vi "CRYCheck Cal Curves for Load or Revert.vi"(8 "In_Out":bool, 9 "Calibration In":T1[](array[typedef]) {"Sens Curve"."Z data" items=["dB", "Lin"]; "Sens Curve"."X data" items=["dB", "Lin"]; "Sens Curve"."Y data" items=["dB", "Lin"]; "Sens Curve"."Z dB ref" format="%.1f"; "Sens Curve"."Z axis" items=["Log", "Lin"]; "Sens Curve"."X dB ref" format="%.1f"; "Sens Curve"."X axis" items=["Log", "Lin"]; "Sens Curve"."Y axis" items=["Log", "Lin"]; "Sens Curve"."Y dB ref" format="%.1f"; "Sens Curve"."Curve"."z" format="%.2f"; "Sens Curve"."Curve"."y" format="%.2f"; "Sens Curve"."Curve"."x" format="%.2f"; "EQ Curve"."Z data" items=["dB", "Lin"]; "EQ Curve"."X data" items=["dB", "Lin"]; "EQ Curve"."Y data" items=["dB", "Lin"]; "EQ Curve"."Z dB ref" format="%.1f"; "EQ Curve"."Z axis" items=["Log", "Lin"]; "EQ Curve"."X dB ref" format="%.1f"; "EQ Curve"."X axis" items=["Log", "Lin"]; "EQ Curve"."Y axis" items=["Log", "Lin"]; "EQ Curve"."Y dB ref" format="%.1f"; "EQ Curve"."Curve"."z" format="%.2f"; "EQ Curve"."Curve"."y" format="%.2f"; "EQ Curve"."Curve"."x" format="%.2f"; "Corr Curve"."Z data" items=["dB", "Lin"]; "Corr Curve"."X data" items=["dB", "Lin"]; "Corr Curve"."Y data" items=["dB", "Lin"]; "Corr Curve"."Z dB ref" format="%.1f"; "Corr Curve"."Z axis" items=["Log", "Lin"]; "Corr Curve"."X dB ref" format="%.1f"; "Corr Curve"."X axis" items=["Log", "Lin"]; "Corr Curve"."Y axis" items=["Log", "Lin"]; "Corr Curve"."Y dB ref" format="%.1f"; "Corr Curve"."Curve"."z" format="%.2f"; "Corr Curve"."Curve"."y" format="%.2f"; "Corr Curve"."Curve"."x" format="%.2f"; "Calibration"."EQ Step size" items=["R10", "R20", "R40", "R80", "User"]; "Calibration"."Corr Step size" items=["R10", "R20", "R40", "R80", "User"]}, 11 "Channel Info_New":T4[](array[typedef]) {"Coupling" items=["Default"=-1, "RSE"=10083, "NRSE"=10078, "Differential"=10106, "Pseudodifferential"=12529]; "term config" items=["Default"=-1, "RSE"=10083, "NRSE"=10078, "Differential"=10106, "Pseudodifferential"=12529]; "Anti-aliasing Factor (%fs)" format="%.2f"}) -> (3 "Calibration Out":T1[](array[typedef]) {"Sens Curve"."Z data" items=["dB", "Lin"]; "Sens Curve"."X data" items=["dB", "Lin"]; "Sens Curve"."Y data" items=["dB", "Lin"]; "Sens Curve"."Z dB ref" format="%.1f"; "Sens Curve"."Z axis" items=["Log", "Lin"]; "Sens Curve"."X dB ref" format="%.1f"; "Sens Curve"."X axis" items=["Log", "Lin"]; "Sens Curve"."Y axis" items=["Log", "Lin"]; "Sens Curve"."Y dB ref" format="%.1f"; "Sens Curve"."Curve"."z" format="%.2f"; "Sens Curve"."Curve"."y" format="%.2f"; "Sens Curve"."Curve"."x" format="%.2f"; "EQ Curve"."Z data" items=["dB", "Lin"]; "EQ Curve"."X data" items=["dB", "Lin"]; "EQ Curve"."Y data" items=["dB", "Lin"]; "EQ Curve"."Z dB ref" format="%.1f"; "EQ Curve"."Z axis" items=["Log", "Lin"]; "EQ Curve"."X dB ref" format="%.1f"; "EQ Curve"."X axis" items=["Log", "Lin"]; "EQ Curve"."Y axis" items=["Log", "Lin"]; "EQ Curve"."Y dB ref" format="%.1f"; "EQ Curve"."Curve"."z" format="%.2f"; "EQ Curve"."Curve"."y" format="%.2f"; "EQ Curve"."Curve"."x" format="%.2f"; "Corr Curve"."Z data" items=["dB", "Lin"]; "Corr Curve"."X data" items=["dB", "Lin"]; "Corr Curve"."Y data" items=["dB", "Lin"]; "Corr Curve"."Z dB ref" format="%.1f"; "Corr Curve"."Z axis" items=["Log", "Lin"]; "Corr Curve"."X dB ref" format="%.1f"; "Corr Curve"."X axis" items=["Log", "Lin"]; "Corr Curve"."Y axis" items=["Log", "Lin"]; "Corr Curve"."Y dB ref" format="%.1f"; "Corr Curve"."Curve"."z" format="%.2f"; "Corr Curve"."Curve"."y" format="%.2f"; "Corr Curve"."Curve"."x" format="%.2f"; "Calibration"."EQ Step size" items=["R10", "R20", "R40", "R80", "User"]; "Calibration"."Corr Step size" items=["R10", "R20", "R40", "R80", "User"]})   [LabVIEW 2013]
uses:
  Typedef Control/CRYCalibration 2DCluster.ctl
  Typedef Control/CRYCalibration Cluster.ctl
  Typedef Control/CRYData Cluster.ctl
  Typedef Control/CRYHardware Channel Info.ctl
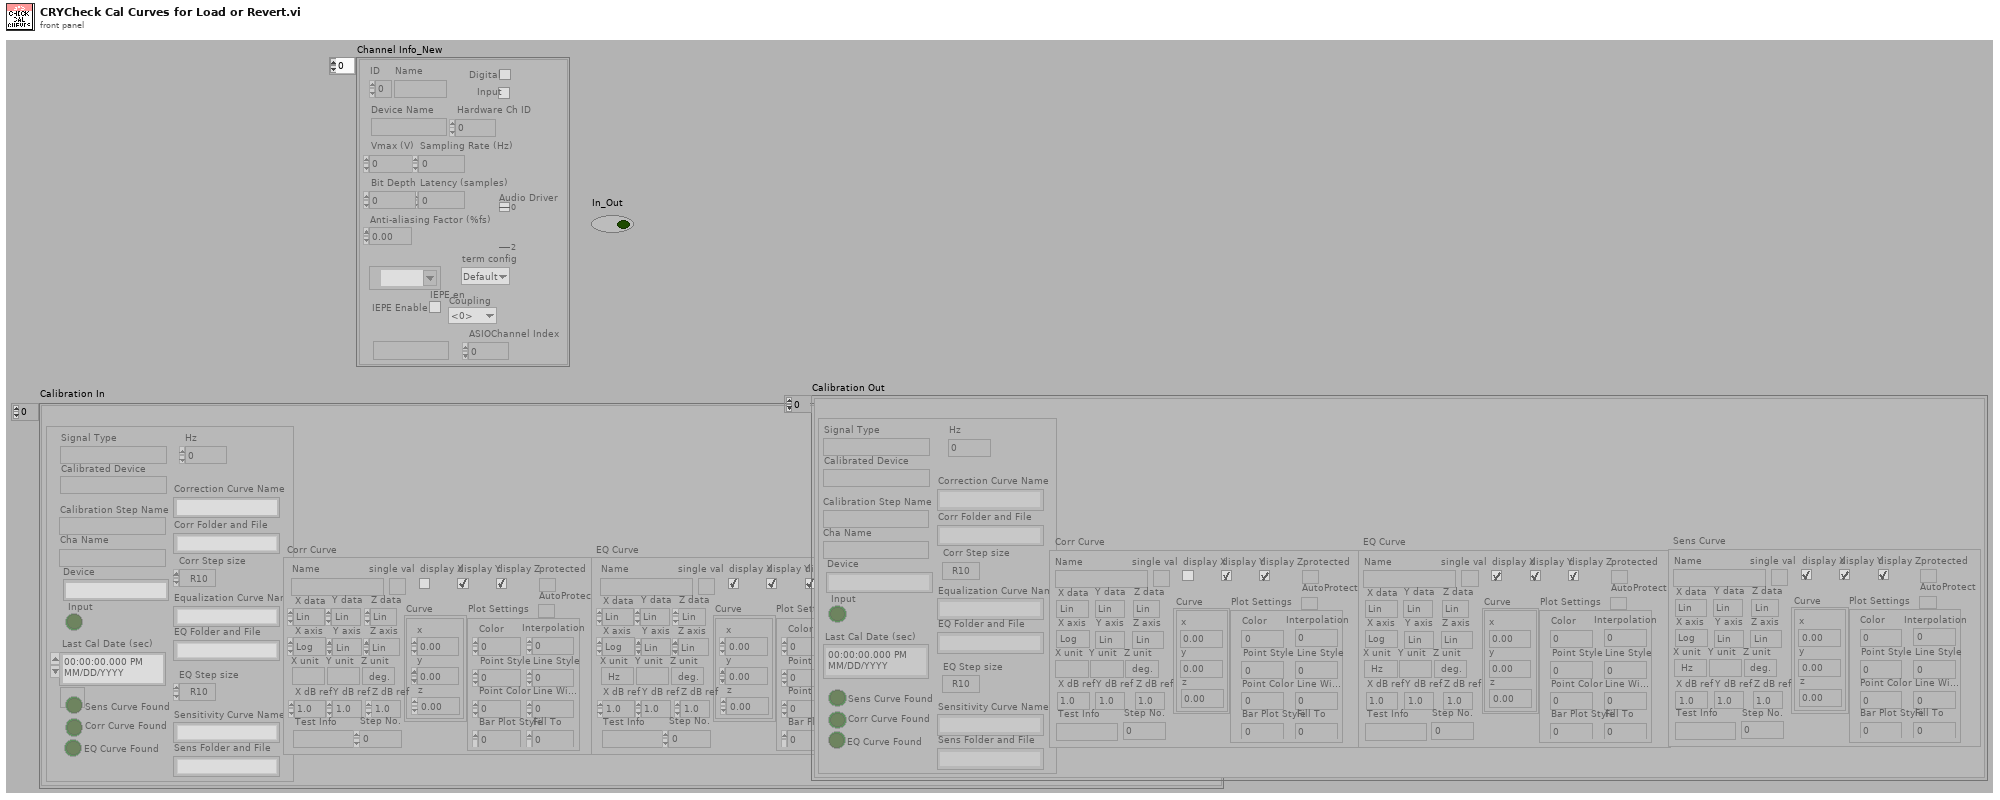
[diagram p1: front panel]
types:
  T1 = typedef "CRYCalibration 2DCluster.ctl" = cluster{"Calibration":T2, "Corr Curve":T3, "EQ Curve":T3, "Sens Curve":T3}
  T2 = typedef "CRYCalibration Cluster.ctl" = cluster{"Calibration Step Name":string, "Device":string, "Correction Curve Name":string, "Equalization Curve Name":string, "Sensitivity Curve Name":string, "Corr Folder and File":string, "EQ Folder and File":string, "Sens Folder and File":string, "Corr Step size":u16, "EQ Step size":u16, "Input":bool, "Last Cal Date (sec)":timestamp, "Cha Name":string, "Corr Curve Found":bool, "EQ Curve Found":bool, "Sens Curve Found":bool, "Signal Type":string, "Calibrated Device":string, "Hz":u32}
  T3 = typedef "CRYData Cluster.ctl" = cluster{"Name":string, "Curve":cluster{"x":dbl, "y":dbl, "z":dbl}[], "X data":u16, "Y data":u16, "Z data":u16, "X axis":u16, "Y axis":u16, "Z axis":u16, "X unit":string, "Y unit":string, "Z unit":string, "X dB ref":dbl, "Y dB ref":dbl, "Z dB ref":dbl, "single val":bool, "protected":bool, "display X":bool, "display Y":bool, "display Z":bool, "Test Info":string, "Step No.":i32, "Plot Settings":cluster{"Color":u32, "Interpolation":u8, "Point Style":u8, "Line Style":u8, "Point Color":u32, "Line Width":u8, "Bar Plot Style":u8, "Fill To":i16}, "AutoProtect":bool}
  T4 = typedef "CRYHardware Channel Info.ctl" = cluster{"ID":i32, "Name":string, "Digital":bool, "Input":bool, "Device Name":string, "Hardware Ch ID":u8, "Vmax (V)":dbl, "Latency (samples)":dbl, "Sampling Rate (Hz)":u32, "Bit Depth":u32, "Anti-aliasing Factor (%fs)":sgl, "DAQmx Channel":tag, "term config":i32, "Coupling":i32, "IEPE en":bool, "ASIOChannel Name":string, "Audio Driver":u16, "ASIOChannel Index":u8}
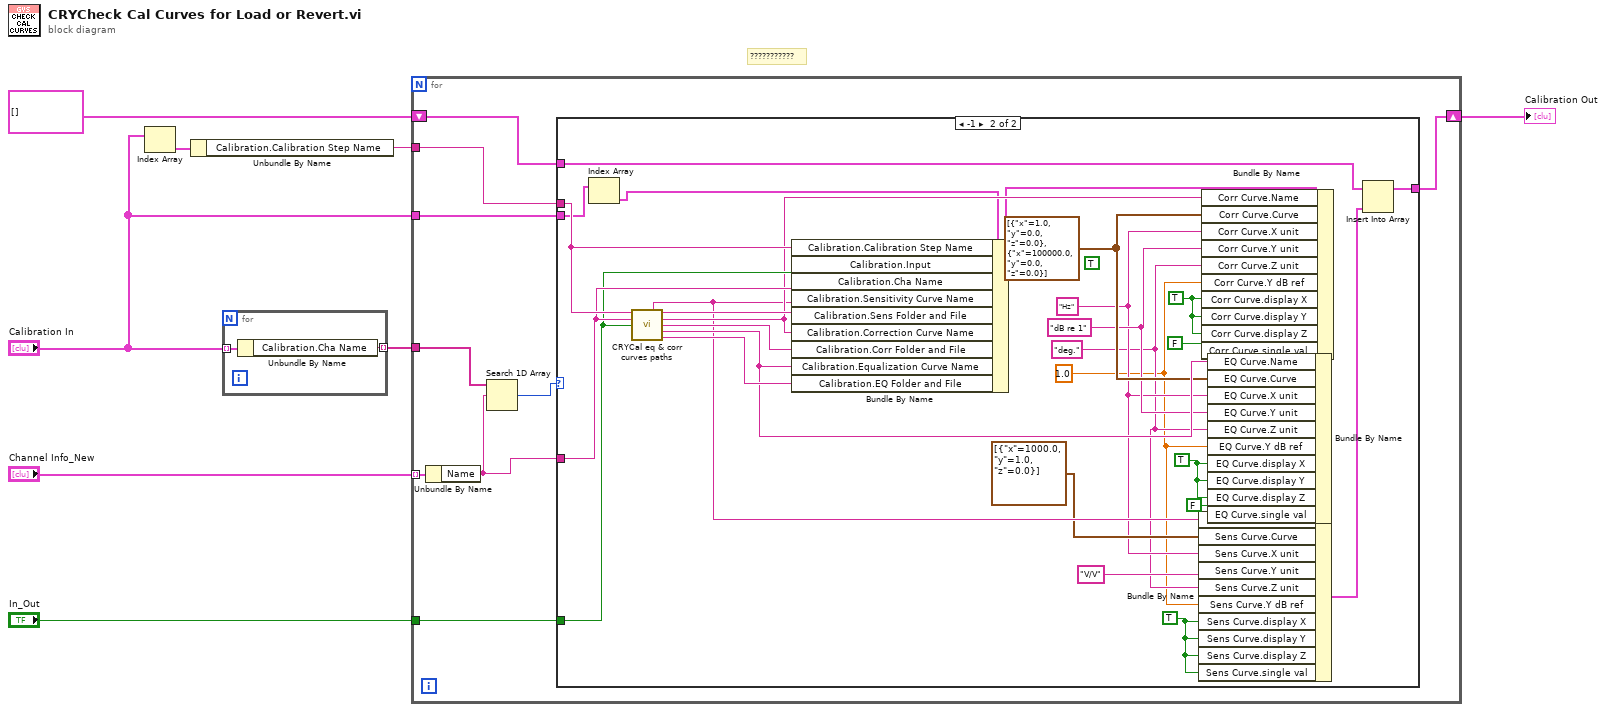
[diagram p0: block diagram]
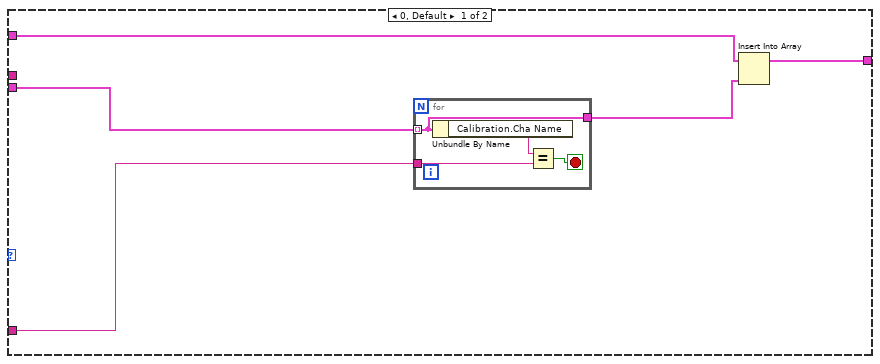
[diagram p2: hidden frame]
diagram:
  # "???????????"
  n1 = Index Array(array="Calibration In") -> (element=w8:T1)  [unwired: 1 in]
  n2 = Unbundle By Name(w8) -> ("Calibration.Calibration Step Name"=w7:string)
  n3 = for {
    tunnel: "Calibration In" -> [w10] mode=indexing
    tunnel: [w9] -> w2 mode=indexing
    n4 = Unbundle By Name(w10) -> ("Calibration.Cha Name"=w9:string)
  }
  n5 = for {
    tunnel: "Channel Info_New" -> [w19] mode=indexing
    tunnel: "Calibration In" -> [w18]
    shift-right: [w16] -> w5
    shift-left: T1[] [] ("Calibration In") -> [w17]
    tunnel: w7 -> [w15]
    tunnel: "In_Out" -> [w14]
    tunnel: w2 -> [w13]
    n6 = Unbundle By Name(w19) -> ("Name"=w12:string)
    n7 = Search 1D Array(1D array=w13, element=w12) -> (index of element=w11:i32)  [unwired: 1 out]
    n8 = case shown="-1" w11 {
      tunnel: w12 -> [w20 w56]
      tunnel: w18 -> [w24 w52]
      tunnel: w17 -> [w23 w51]
      tunnel: [w21 w50] -> w16
      tunnel: w15 -> [_ w57]
      tunnel: w14 -> [_ w55]
      frame 0, Default {
        n9 = for {
          tunnel: w24 -> [w25] mode=indexing
          tunnel: w20 -> [w28]
          tunnel: [w25] -> w22
          stop <- w26 stop-if-true
          n10 = Unbundle By Name(w25) -> ("Calibration.Cha Name"=w27:string)
          n11 = Equal?(x=w27, y=w28) -> (x = y?=w26:bool)
        }
        n12 = Insert Into Array(array=w23, new element=w22) -> (w21:T1[])  [unwired: 1 in]
      }
      frame -1 {
        w33 = TRUE ("Sens Curve.display X")
        w41 = TRUE ("EQ Curve.display X")
        w47 = TRUE ("Corr Curve.display X")
        w34 = 1.0 ("EQ Curve.Y dB ref")
        w35 = "deg." ("Corr Curve.Z unit")
        w42 = "dB re 1" ("Corr Curve.Y unit")
        w36 = "Hz" ("Corr Curve.X unit")
        w43 = cluster{"x":dbl, "y":dbl, "z":dbl}[] [{"x"=1.0, "y"=0.0, "z"=0.0}, {"x"=100000.0, "y"=0.0, "z"=0.0}] ("Corr Curve.Curve")
        (unwired) TRUE ("Sens Curve.single val")
        n13 = Index Array(array=w52) -> (element=w45:T1)  [unwired: 1 in]
        n14 = call "CRYCal eq & corr curves paths.vi"("Calibrated Device Name"=w57, "Channel Name"=w56, "In_Out"=w55) -> ("Sens Currve Name"=w39:string, "Sens Curve File"=w54:string, "Corr Curve Name"=w48:string, "Corr Curve File"=w49:string, "EQ Curve Name"=w44:string, "EQ Curve File"=w53:string)  [unwired: 7 out]
        n15 = Bundle By Name(cluster=w45, "Calibration.Calibration Step Name"=w57, "Calibration.Input"=w55, "Calibration.Cha Name"=w56, "Calibration.Sensitivity Curve Name"=w39, "Calibration.Sens Folder and File"=w54, "Calibration.Correction Curve Name"=w48, "Calibration.Corr Folder and File"=w49, "Calibration.Equalization Curve Name"=w44, "Calibration.EQ Folder and File"=w53) -> (w32:T1)
        n16 = Bundle By Name(cluster=w32, "Corr Curve.Name"=w48, "Corr Curve.Curve"=w43, "Corr Curve.X unit"=w36, "Corr Curve.Y unit"=w42, "Corr Curve.Z unit"=w35, "Corr Curve.Y dB ref"=w34, "Corr Curve.display X"=w47, "Corr Curve.display Y"=w47, "Corr Curve.display Z"=w47, "Corr Curve.single val"=FALSE) -> (w31:T1)
        n17 = Bundle By Name(cluster=w31, "EQ Curve.Name"=w44, "EQ Curve.Curve"=w43, "EQ Curve.X unit"=w36, "EQ Curve.Y unit"=w42, "EQ Curve.Z unit"=w35, "EQ Curve.Y dB ref"=w34, "EQ Curve.display X"=w41, "EQ Curve.display Y"=w41, "EQ Curve.display Z"=w41, "EQ Curve.single val"=FALSE) -> (w30:T1)
        n18 = Bundle By Name(cluster=w30, "Sens Curve.Name"=w39, "Sens Curve.Curve"=cluster{"x":dbl, "y":dbl, "z":dbl}[] [{"x"=1000.0, "y"=1.0, "z"=0.0}], "Sens Curve.X unit"=w36, "Sens Curve.Y unit"="V/V", "Sens Curve.Z unit"=w35, "Sens Curve.Y dB ref"=w34, "Sens Curve.display X"=w33, "Sens Curve.display Y"=w33, "Sens Curve.display Z"=w33, "Sens Curve.single val"=w33) -> (w29:T1)
        n19 = Insert Into Array(array=w51, new element=w29) -> (w50:T1[])  [unwired: 1 in]
      }
    }
  }
  "Calibration Out" <- w5
